vi "ReadConfigIniCluster.vi"(0 "更随产品型号变更？":bool, 1 "ConfigFlieName":string="DAQSetting.ini收参数.ini", 2 "ConfigOut":variant, 3 "ProductName":string="产品名称XXX", 5 "error in (no error)":errorcluster caption="错误输入（无错误）", 6 "根路径":path) -> (16 "ConfigOut":variant, 19 "error out":errorcluster caption="错误输出")   [LabVIEW 2020]
uses:
  <vilib>/Utility/config.llb/NI_LVConfig.lvlib
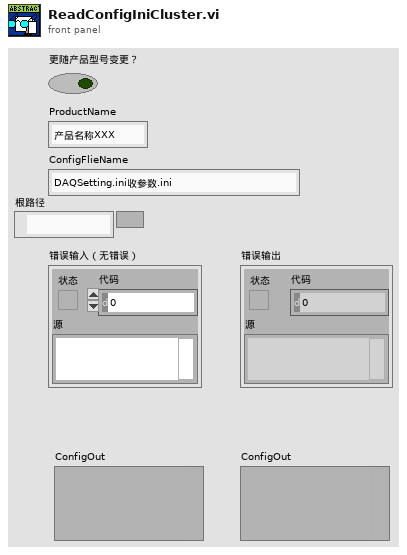
[diagram p1: front panel]
types:
  T1 = typedef "NI_LVConfig.lvlib/Config Data RefNum.ctl" = refnum<k1>
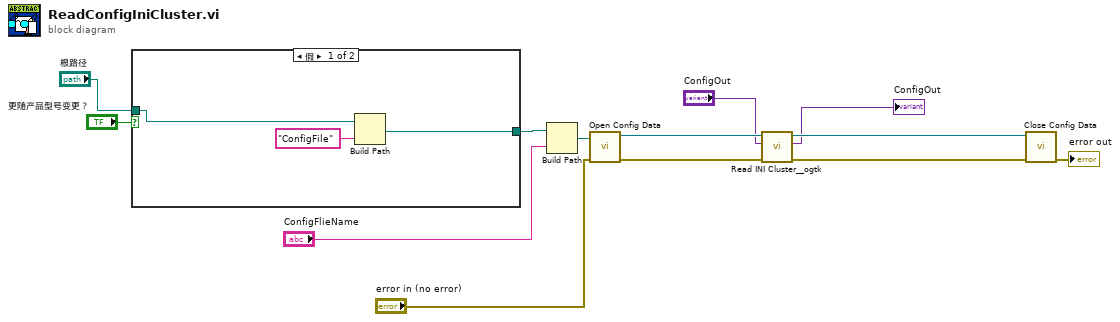
[diagram p0: block diagram]
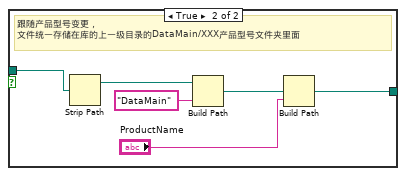
[diagram p2: hidden frame]
diagram:
  n1 = case shown="假" "更随产品型号变更？" {
    tunnel: [w15 w19] -> w10
    tunnel: "根路径" -> [w14 w17]
    frame False {
      n2 = Build Path(base path=w14, name or relative path="ConfigFile" ("ConfigFlieFolderName")) -> (appended path=w15:path)
    }
    frame True {
      # "跟随产品型号变更，\n文件统一存储在库的上一级目录的DataMain/XXX产品型号文件夹里面"
      n3 = Strip Path(path=w17) -> (stripped path=w21:path)  [unwired: 1 out]
      n4 = Build Path(base path=w21, name or relative path="DataMain" ("ConfigFlieFolderName")) -> (appended path=w20:path)
      n5 = Build Path(base path=w20, name or relative path="ProductName") -> (appended path=w19:path)
    }
  }
  n6 = Build Path(base path=w10, name or relative path="ConfigFlieName") -> (appended path=w9:path)
  n7 = call <vilib>:"Open Config Data.vi"("error in (no error)"="error in (no error)", "configuration file path"=w9) -> ("error out"=w6:errorcluster, "refnum"=w5:T1)  [unwired: 7 in, 1 out]
  n8 = call <userlib>:"Read INI Cluster__ogtk.vi"("error in (no error)"=w6, "INI Fomatted Cluster Type"="ConfigOut", "refnum"=w5) -> ("error out"=w12:errorcluster, "INI Fomatted Cluster"=→"ConfigOut":variant, "dup refnum"=w13:T1)  [unwired: 4 in, 2 out]
  n9 = call <vilib>:"Close Config Data.vi"("error in (no error)"=w12, "refnum"=w13) -> ("error out"=→"error out":errorcluster)  [unwired: 8 in, 1 out]
